vi "State Machine logging.vi"(0 "reference in":refnum<class "Generic Utilities.lvclass">, 5 "error in (no error)":errorcluster, 7 "Latest State":string) -> (14 "reference out":refnum<class "Generic Utilities.lvclass">, 19 "error out":errorcluster)   [LabVIEW 2020, in "Generic Utilities.lvclass"]
uses:
  Generic Utilities.lvclass
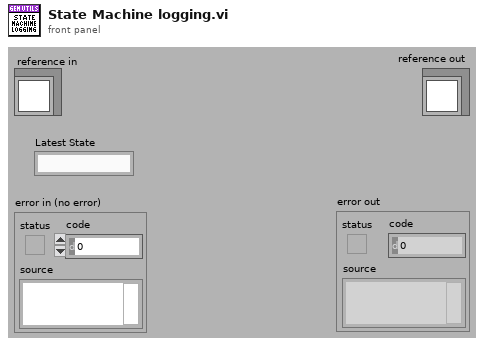
[diagram p1: front panel]
types:
  T1 = enum16{"open", "replace", "create", "open or create", "replace or create", "replace or create with confirmation"}
  T2 = typedef "Generic Utilities.lvclass/ObjectAttributes.ctl" = cluster{"GUI Parameters":T3, "State Machine Control":cluster{"Timeout":i32, "State Queue":string[], "State History":string[], "State History Length":i32}, "Logging File Path":path, "OBJ not a refnum?":bool, "Timer Start":timestamp, "FP Refnums":T4}
  T3 = typedef "Generic Utilities.lvclass/GUI Parameters.ctl" = cluster{"Application Name":string, "GUI VI Ref":refnum<vi>, "Close Panel?":bool, "Message Window ref":refnum<vi>, "Version #":string}
  T4 = typedef "Generic Utilities.lvclass/FP Refnums.ctl" = cluster{"Panel refnum":refnum<vi>, "Control Labels":string[], "Refnums":refnum<vi>[]}
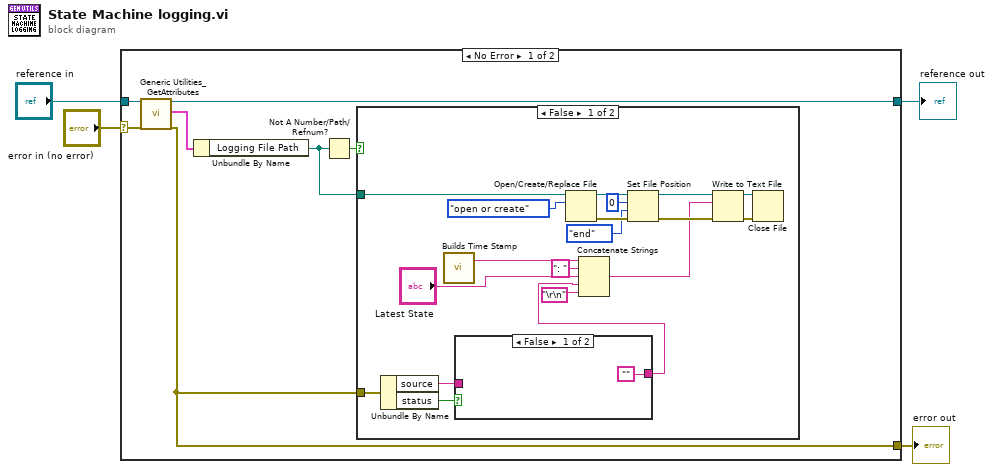
[diagram p0: block diagram]
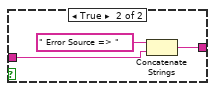
[diagram p2: hidden frame]
diagram:
  n1 = case shown="No Error" "error in (no error)" {
    selector: "error in (no error)" -> [w11 w36]
    tunnel: [w5 w36] -> w3
    tunnel: [w10 w35] -> w1
    tunnel: "reference in" -> [w8 w35]
    frame No Error {
      n2 = call "Generic Utilities_GetAttributes.vi"("reference in"=w8, "error in (no error)"=w11) -> ("reference out"=w10:refnum<class "Generic Utilities.lvclass">, "attributes"=w9:T2, "error out"=w5:errorcluster)  [unwired: 14 in, 1 out]
      n3 = Unbundle By Name(w9) -> ("Logging File Path"=w6:path)
      n4 = Not A Number/Path/Refnum?(number/path/refnum=w6) -> (NaN/Path/Refnum?=w7:bool)
      n5 = case shown="False" w7 {
        tunnel: w6 -> [w17 _]
        tunnel: w5 -> [w15 _]
        frame False {
          n6 = Unbundle By Name(w15) -> ("source"=w13:string, "status"=w14:bool)
          n7 = call "Builds Time Stamp.vi"() -> ("TimeStamp"=w18:string)  [unwired: 19 in]
          n8 = case shown="False" w14 {
            tunnel: w13 -> [_ w33]
            tunnel: ["" w32] -> w12
            frame False {
            }
            frame True {
              n9 = Concatenate Strings(" Error Source => ", w33) -> (w32:string)
            }
          }
          n10 = Open/Create/Replace File(file path (use dialog)=w17, operation (0:open)=T1."open or create") -> (refnum out=w26:refnum<file>, error out=w27:errorcluster)  [unwired: 4 in, 1 out]
          n11 = Concatenate Strings(w18, ": " ("string"), "Latest State", w12, "\r\n") -> (w20:string)
          n12 = Set File Position(offset (in bytes) (0)=i64 0, refnum=w26, from (0:start)=enum16{"start", "end", "current"}."end", error in=w27) -> (refnum out=w28:refnum<file>, error out=w29:errorcluster)
          n13 = Write to Text File(file (use dialog)=w28, text=w20, error in=w29) -> (refnum out=w22:refnum<file>, error out=w21:errorcluster)  [unwired: 1 in, 1 out]
          n14 = Close File(refnum=w22, error in=w21) -> ()  [unwired: 2 out]
        }
        frame True {
          # "There are no file path, so do NOT logging."
        }
      }
    }
    frame Error {
    }
  }
  "error out" <- w3
  "reference out" <- w1
